vi "4-and.vi"(1 "Boolean 4":bool, 2 "Boolean 3":bool, 3 "Boolean 2":bool, 4 "Boolean":bool) -> (0 "Boolean 5":bool)   [LabVIEW 2018]
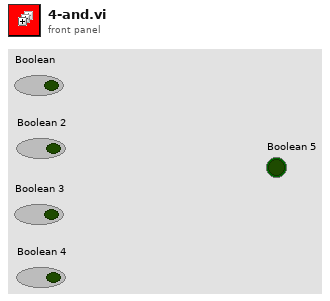
[diagram p1: front panel]
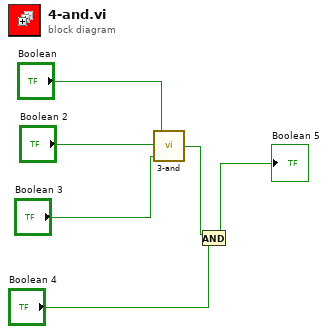
[diagram p0: block diagram]
diagram:
  n1 = call "3-and.vi"("Boolean 2"="Boolean 3", "Boolean 4"="Boolean 2", "Boolean 3"="Boolean") -> ("Boolean"=w3:bool)
  n2 = And(x=w3, y="Boolean 4") -> (x .and. y?=→"Boolean 5":bool)
